vi "다중Queue입력_Test.vi"() -> ()   [LabVIEW 2023]
panel:
  out "부분이 삭제된 배열":string[][](array[string])
  out "삭제된 부분":string[][](array[string])
  out "원소":string[][](array[string])
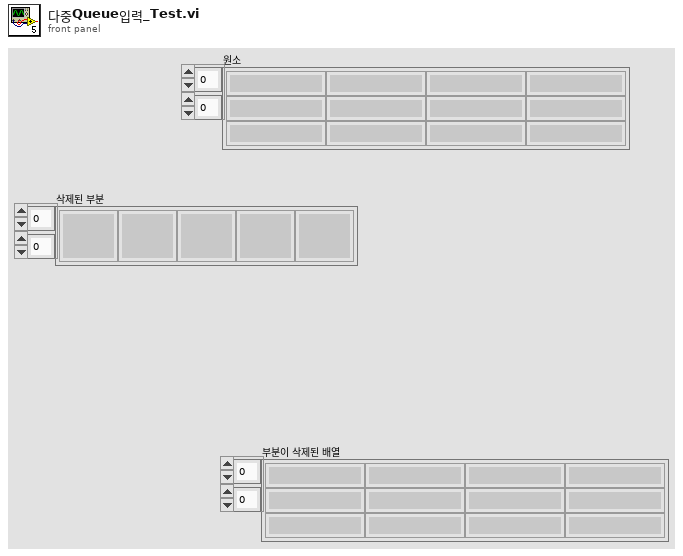
[diagram p1: front panel]
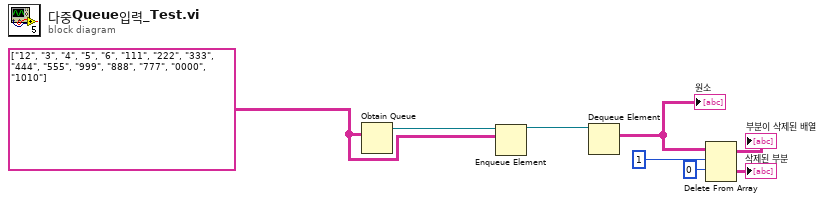
[diagram p0: block diagram]
diagram:
  w6 = string[][] [["12", "3", "4", "5", "6"], ["111", "222", "333", "444", "555"], ["999", "888", "777", "0000", "1010"]] ("이름(이름없음)")
  n1 = Obtain Queue(element data type=w6) -> (queue out=w8:refnum<queue>)  [unwired: 4 in, 2 out]
  n2 = Enqueue Element(queue=w8, element=w6) -> (queue out=w7:refnum<queue>)  [unwired: 2 in, 2 out]
  n3 = Dequeue Element(queue=w7) -> (element=w5:string[][])  [unwired: 2 in, 3 out]
  "원소" <- w5
  n4 = Delete From Array(array=w5, length=1 ("길이"), index (row)=0 ("인덱스 (행)")) -> (deleted portion=→"삭제된 부분":string[][], array with subset deleted=→"부분이 삭제된 배열":string[][])  [unwired: 1 in]
